vi "RCV CAN data FD.vi"() -> ()   [LabVIEW 2016]
doc: "This is a practical example of CAN_READ_FD.\nOn the left hand side of the BD is a disabled code section. One can enable this to log CAN data.\nThe potput of this disabled code segment is the error cluster.\nThan the selected channel will be initiatlized.\nOnce the initialisation is OK a timed while loop will be executed until CAN_READ_FD will signal an error.\nInside of the while loop is the CAN_READ_FD function.\nBuilding up an array of CAN mesages and timestamps is done while this loop executes.\nOnly the last message witch is naturaly empty, because the receive queue is empty, will be ignored.\nThe result is an array of received CAN messages."
uses:
  CAN Communication.llb/TPCANHandle.ctl
  CAN Communication.llb/TPCANTimestampFD.ctl
  CAN Communication.llb/CAN MSG Cluster.ctl
  CAN Communication.llb/TPCANParameter.ctl
  <vilib>/Platform/TimedLoop/XDataNode/timing_clust.ctl
  <vilib>/Platform/TimedLoop/XDataNode/nitl_modes.ctl
  <vilib>/Platform/TimedLoop/XDataNode/wakeup.ctl
  CAN Communication.llb/PCAN Get CHANNEL CONDITION.vi
  <vilib>/Platform/TimedLoop/XDataNode/XDataNode.xnode
  <vilib>/Platform/TimedLoop/XDataNode/XDNodeRunTimeDep.lvlib
  D:/Persoenliche_Daten/LabVIEW/VI.LIB/Peak/LV_basic FD Auslieferung/.LV Win32 VIs/Controls/LOG config.ctl
  D:/Persoenliche_Daten/LabVIEW/VI.LIB/Peak/LV_basic FD Auslieferung/.LV Win32 VIs/VIs/Set Value/PCAN Set LOG CONFIGURE.vi
  D:/Persoenliche_Daten/LabVIEW/VI.LIB/Peak/LV_basic FD Auslieferung/.LV Win32 VIs/VIs/Set Value/PCAN Set LOG LOCATION.vi
panel:
  out "TPCANMessageType out Strings":string
  out "CAN Data out":T1[](array[typedef]) {"MSG type" format="%x"; "ID" format="%.0x"}
  out "CAN Timestamp data out":T2[](array[typedef]) format="%x"
  in  "Release all channels first":bool
  in  "TPCANHandle":T3=enum."PCAN_USBBUS1  0x51"
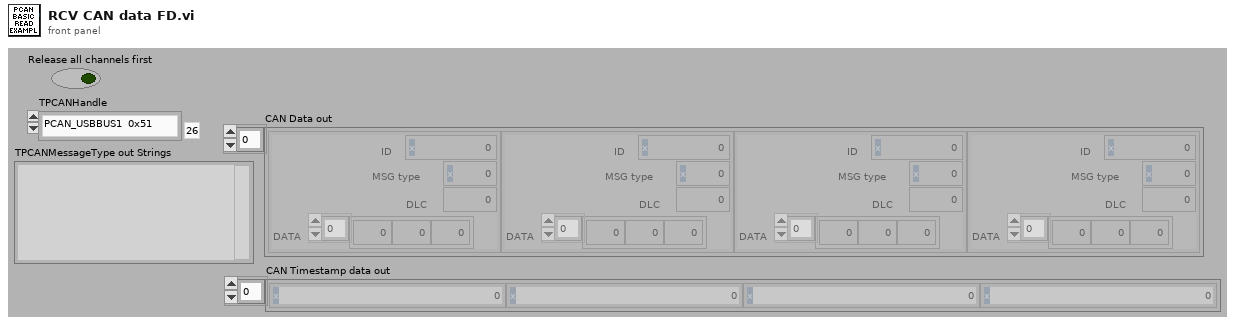
[diagram p1: front panel]
types:
  T1 = typedef "CAN MSG Cluster.ctl" = cluster{"ID":u32, "MSG type":u8, "DLC":u8, "DATA":u8[]}
  T2 = typedef "TPCANTimestampFD.ctl" = u64
  T3 = typedef "TPCANHandle.ctl" = enum16{"PCAN_NONEBUS  0x000", "PCAN_ISABUS1  0x21", "PCAN_ISABUS2  0x22", "PCAN_ISABUS3  0x23", "PCAN_ISABUS4  0x24", "PCAN_ISABUS5  0x25", "PCAN_ISABUS6  0x26", "PCAN_ISABUS7  0x27", "PCAN_ISABUS8  0x28", "PCAN_DNGBUS1  0x31", "PCAN_PCIBUS1  0x41", "PCAN_PCIBUS1  0x42", "PCAN_PCIBUS1  0x43", "PCAN_PCIBUS1  0x44", "PCAN_PCIBUS1  0x45", "PCAN_PCIBUS1  0x46", "PCAN_PCIBUS1  0x47", "PCAN_PCIBUS1  0x48", "PCAN_PCIBUS1  0x409", "PCAN_PCIBUS1  0x40A", "PCAN_PCIBUS1  0x40B", "PCAN_PCIBUS1  0x40C", "PCAN_PCIBUS1  0x40D", "PCAN_PCIBUS1  0x40E", "PCAN_PCIBUS1  0x40F", "PCAN_PCIBUS1  0x410", "PCAN_USBBUS1  0x51", "PCAN_USBBUS2  0x52", "PCAN_USBBUS3  0x53", "PCAN_USBBUS4  0x54", "PCAN_USBBUS5  0x55", "PCAN_USBBUS6  0x56", "PCAN_USBBUS7  0x57", "PCAN_USBBUS8  0x58", "PCAN_USBBUS9  0x509", "PCAN_USBBUS10  0x50A", "PCAN_USBBUS11  0x50B", "PCAN_USBBUS12  0x50C", "PCAN_USBBUS13  0x50D", "PCAN_USBBUS14  0x50E", "PCAN_USBBUS15  0x50F", "PCAN_USBBUS16  0x510", "PCAN_PCCBUS1  0x61", "PCAN_PCCBUS2  0x62", "PCAN_LANBUS1  0x801", "PCAN_LANBUS2  0x802", "PCAN_LANBUS3  0x803", "PCAN_LANBUS4  0x804", "PCAN_LANBUS5  0x805", "PCAN_LANBUS6  0x806", "PCAN_LANBUS7  0x807", "PCAN_LANBUS8  0x808", "PCAN_LANBUS9  0x809", "PCAN_LANBUS10  0x80A", "PCAN_LANBUS11  0x80B", "PCAN_LANBUS12  0x80C", "PCAN_LANBUS13  0x80D", "PCAN_LANBUS14  0x80E", "PCAN_LANBUS15  0x80F", "PCAN_LANBUS16  0x810"}
  T4 = typedef "TPCANParameter.ctl" = enum8{"Not Available", "PCAN device number", "PCAN 5-volt power", "PCAN receive event", "PCAN message filter", "PCAN API version", "PCAN channel version", "PCAN busoff autoreset", "PCAN listen-only", "PCAN log location", "PCAN log status", "PCAN log configure", "PCAN log text", "PCAN channel condition", "PCAN hardware name", "PCAN_RECEIVE_STATUS", "PCAN_CONTROLLER_NUMBER", "PCAN_TRACE_LOCATION ", "PCAN_TRACE_STATUS", "PCAN_TRACE_SIZE", "PCAN_TRACE_CONFIGURE", "PCAN_CHANNEL_IDENTIFYING", "PCAN_CHANNEL_FEATURES", "PCAN_SPEED_ADAPTING", "PCAN_BITRATE_INFO", "PCAN_BITRATE_INFO_FD", "PCAN_BUSSPEED_NOMINAL", "PCAN_BUSSPEED_DATA", "PCAN_IP_ADDRESS", "PCAN_LAN_SERVICE_STATUS", "PCAN_ALLOW_STATUS_FRAMES", "PCAN_ALLOW_RTR_FRAMES", "PCAN_ALLOW_ERROR_FRAMES", "PCAN_INTERFRAME_DELAY", "PCAN_ACCEPTANCE_FILTER_11BIT", "PCAN_ACCEPTANCE_FILTER_29BIT", "PCAN_IO_DIGITAL_CONFIGURATION", "PCAN_IO_DIGITAL_VALUE", "PCAN_IO_DIGITAL_SET", "PCAN_IO_DIGITAL_CLEAR", "PCAN_IO_ANALOG_VALUE"}
  T5 = typedef "PCAN BASIC FD.lvlib/LOG config.ctl" = u32
  T6 = typedef "PCAN BASIC FD.lvlib/TPCANHandle.ctl" = enum16{"PCAN_NONEBUS  0x000", "PCAN_ISABUS1  0x21", "PCAN_ISABUS2  0x22", "PCAN_ISABUS3  0x23", "PCAN_ISABUS4  0x24", "PCAN_ISABUS5  0x25", "PCAN_ISABUS6  0x26", "PCAN_ISABUS7  0x27", "PCAN_ISABUS8  0x28", "PCAN_DNGBUS1  0x31", "PCAN_PCIBUS1  0x41", "PCAN_PCIBUS1  0x42", "PCAN_PCIBUS1  0x43", "PCAN_PCIBUS1  0x44", "PCAN_PCIBUS1  0x45", "PCAN_PCIBUS1  0x46", "PCAN_PCIBUS1  0x47", "PCAN_PCIBUS1  0x48", "PCAN_PCIBUS1  0x409", "PCAN_PCIBUS1  0x40A", "PCAN_PCIBUS1  0x40B", "PCAN_PCIBUS1  0x40C", "PCAN_PCIBUS1  0x40D", "PCAN_PCIBUS1  0x40E", "PCAN_PCIBUS1  0x40F", "PCAN_PCIBUS1  0x410", "PCAN_USBBUS1  0x51", "PCAN_USBBUS2  0x52", "PCAN_USBBUS3  0x53", "PCAN_USBBUS4  0x54", "PCAN_USBBUS5  0x55", "PCAN_USBBUS6  0x56", "PCAN_USBBUS7  0x57", "PCAN_USBBUS8  0x58", "PCAN_USBBUS9  0x509", "PCAN_USBBUS10  0x50A", "PCAN_USBBUS11  0x50B", "PCAN_USBBUS12  0x50C", "PCAN_USBBUS13  0x50D", "PCAN_USBBUS14  0x50E", "PCAN_USBBUS15  0x50F", "PCAN_USBBUS16  0x510", "PCAN_PCCBUS1  0x61", "PCAN_PCCBUS2  0x62", "PCAN_LANBUS1  0x81", "PCAN_LANBUS2  0x82", "PCAN_LANBUS3  0x83", "PCAN_LANBUS4  0x84", "PCAN_LANBUS5  0x85", "PCAN_LANBUS6  0x86", "PCAN_LANBUS7  0x87", "PCAN_LANBUS8  0x88", "PCAN_LANBUS9  0x809", "PCAN_LANBUS10  0x80A", "PCAN_LANBUS11  0x80B", "PCAN_LANBUS12  0x80C", "PCAN_LANBUS13  0x80D", "PCAN_LANBUS14  0x80E", "PCAN_LANBUS15  0x80F", "PCAN_LANBUS16  0x810"}
  T7 = typedef "Channel Availability.ctl" = enum16{"PCAN_CHANNEL_UNAVAILABLE", "PCAN_CHANNEL_AVAILABLE", "PCAN_CHANNEL_OCCUPIED"}
  T8 = typedef "XDNodeRunTimeDep.lvlib/timing_clust.ctl" = cluster{"Expected End [f-1]":u64, "Actual End [f-1]":u64, "Finished Late? [f-1]":bool, "Expected End [i-1]":u64, "Actual End [i-1]":u64, "Finished Late? [i-1]":bool, "Expected Start [i]":u64, "Actual Start [i]":u64, "Expected Start [f]":u64, "Actual Start [f]":u64, "Source Name":string, "Structure Name":string, "Period":i64, "Deadline":i64, "Offset":i64, "Start":i64, "Priority":i32, "Timeout":i32, "Mode":T9, "Wakeup Reason":T10, "Error":errorcluster, "Source Type":string, "Secondary Source Type":string, "Global End Time":u64, "Global Start Time":u64, "Frame Duration":u64, "Iteration Duration":u64, "Assigned CPU":i32, "I/O Scan Engine Mode":u32}
  T9 = typedef "XDNodeRunTimeDep.lvlib/nitl_modes.ctl" = enum32{"No Change", "Process missed periods, maintain original phase", "Discard missed periods, maintain original phase", "Process missed periods, ignore original phase", "Discard missed periods, ignore original phase"}
  T10 = typedef "XDNodeRunTimeDep.lvlib/wakeup.ctl" = enum32{"Normal", "Aborted", "Asynchronous wakeup", "Timing source error", "Timed loop error", "Timeout"}
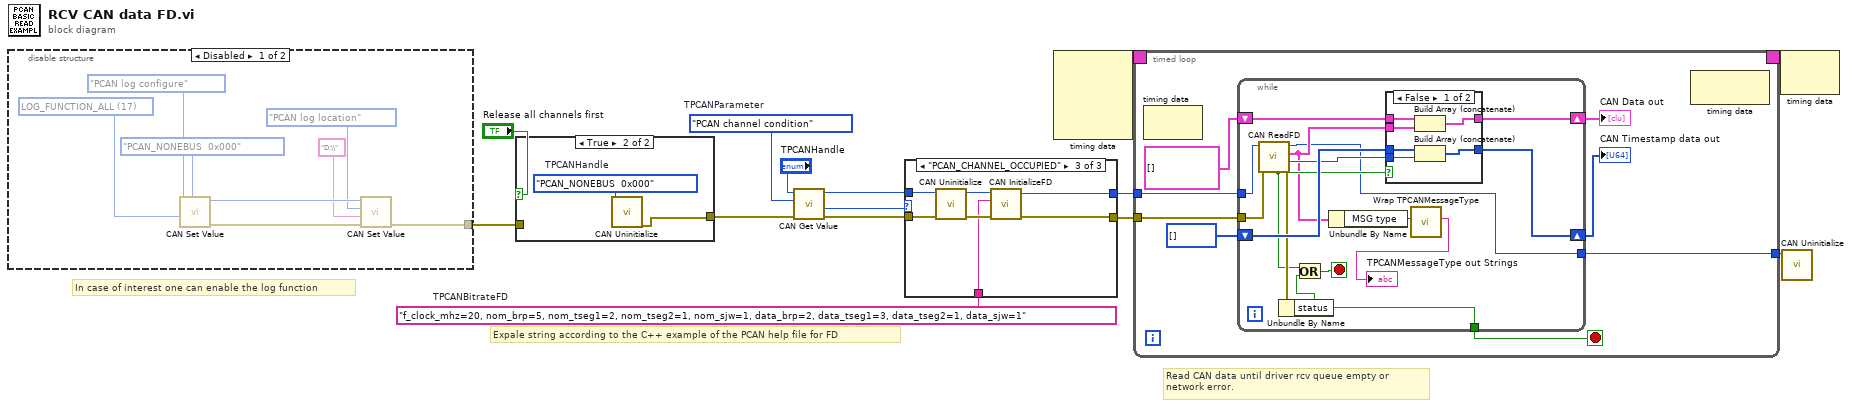
[diagram p0: block diagram]
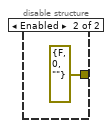
[diagram p3: hidden frame]
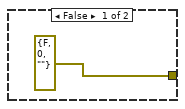
[diagram p4: hidden frame]
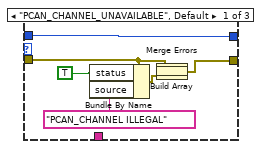
[diagram p5: hidden frame]
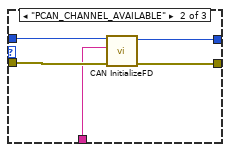
[diagram p6: hidden frame]
diagram:
  w9 = "f_clock_mhz=20, nom_brp=5, nom_tseg1=2, nom_tseg2=1, nom_sjw=1, data_brp=2, data_tseg1=3, data_tseg2=1, data_sjw=1"  # TPCANBitrateFD
  w14 = TPCANParameter."PCAN channel condition"  # TPCANParameter
  # "In case of interest one can enable the log function"
  # "Read CAN data until driver rcv queue empty or\nnetwork error."
  # "Expale string according to the C++ example of the PCAN help file for FD"
  n1 = disable-structure shown="Disabled" {
    disable-tunnel: [w15 errorcluster {"status"=FALSE, "code"=0, "source"=""} ("error out")] -> w6
    frame Disabled {
      w16 = T5 17 items=["LOG_FUNCTION_DEFAULT", "LOG_FUNCTION_ENTRY", "LOG_FUNCTION_PARAMETERS", "Not available", "LOG_FUNCTION_LEAVE", "Not available", "Not available", "Not available", "LOG_FUNCTION_WRITE", "Not available", "Not available", "Not available", "Not available", "Not available", "Not available", "Not available", "LOG_FUNCTION_READ", "LOG_FUNCTION_ALL"] ("LOG config")
      n2 = call-poly "CAN Set Value.vi"("LOG config"=w16, "TPCANParameter"=TPCANParameter."PCAN log configure", "TPCANHandle"=TPCANHandle."PCAN_NONEBUS  0x000") -> ("error out"=w21:errorcluster, "TPCANHandle out"=w20:T6)  [unwired: 7 in]
      n3 = call-poly "CAN Set Value.vi"("error in (no error)"=w21, "LOG LOCATION (path string)"="D:\\", "Parameter"=TPCANParameter."PCAN log location", "TPCANHandle"=w20) -> ("error out"=w15:errorcluster)  [unwired: 6 in, 1 out]
    }
    frame Enabled {
    }
  }
  n4 = case shown="True" "Release all channels first" {
    tunnel: [errorcluster {"status"=FALSE, "code"=0, "source"=""} ("error out") w26] -> w7
    tunnel: w6 -> [_ _]
    frame False {
    }
    frame True {
      w25 = TPCANHandle."PCAN_NONEBUS  0x000"  # TPCANHandle
      n5 = call "CAN Uninitialize.vi"("TPCANHandle"=w25) -> ("error out"=w26:errorcluster)  [unwired: 8 in, 2 out]
    }
  }
  n6 = call-poly "CAN Get Value.vi"("error in (no error)"=w7, "TPCANParameter"=w14, "TPCANHandle"="TPCANHandle") -> ("error out"=w12:errorcluster, "Channel condition"=w11:T7, "TPCANHandle out"=w13:T3)  [unwired: 6 in]
  n7 = case shown="\"PCAN_CHANNEL_OCCUPIED\"" w11 {
    tunnel: [w32 w38 w42] -> w3
    tunnel: w13 -> [w33 w37 w44]
    tunnel: w12 -> [w31 w36 w45]
    tunnel: [w33 w35 w40] -> w2
    tunnel: w9 -> [_ w34 w39]
    frame "PCAN_CHANNEL_UNAVAILABLE", Default {
      n8 = Bundle By Name(cluster=w31, "status"=TRUE, "source"="PCAN_CHANNEL ILLEGAL") -> (w28:errorcluster)
      n9 = Build Array(w31, w28) -> (w27:errorcluster[])
      n10 = Merge Errors(w27) -> (w32:errorcluster)
    }
    frame "PCAN_CHANNEL_AVAILABLE" {
      n11 = call "CAN InitializeFD.vi"("error in (no error)"=w36, "TPCANBitrateFD"=w34, "TPCANHandle"=w37) -> ("error out"=w38:errorcluster, "TPCANHandle out"=w35:T3)  [unwired: 5 in, 2 out]
    }
    frame "PCAN_CHANNEL_OCCUPIED" {
      n12 = call "CAN Uninitialize.vi"("error in (no error)"=w45, "TPCANHandle"=w44) -> ("error out"=w43:errorcluster, "TPCANHandle out"=w41:T3)  [unwired: 7 in, 1 out]
      n13 = call "CAN InitializeFD.vi"("error in (no error)"=w43, "TPCANBitrateFD"=w39, "TPCANHandle"=w41) -> ("error out"=w42:errorcluster, "TPCANHandle out"=w40:T3)  [unwired: 5 in, 2 out]
    }
  }
  n14 = node-c288() -> (w5:T8)  [unwired: 4 in]
  n15 = timed-loop {
    timing: w5 -> [_]
    timing-out: [_] -> w4
    tunnel: w2 -> [w53]
    tunnel: w3 -> [w52]
    tunnel: [w46] -> w1
    stop <- w51 stop-if-true
    n16 = node-c288() -> ()  [unwired: 1 in, 1 out]
    n17 = while {
      tunnel: w53 -> [w62]
      tunnel: w52 -> [w61]
      tunnel: [w67] -> w51
      shift-right: [w65] -> w50
      shift-left: T1[] [] -> [w66]
      shift-right: [w63] -> w47
      shift-left: u64[] [] -> [w64]
      tunnel: [w54] -> w46
      stop <- w68 stop-if-true
      n18 = call "CAN ReadFD.vi"("error in (no error)"=w61, "TPCANHandle"=w62) -> ("error out"=w59:errorcluster, "TPCANTimestamp out"=w60:T2, "CAN_Message out"=w55:T1, "TPCANHandle out"=w54:T3, "rcv queue empty"=w58:bool)  [unwired: 5 in]
      n19 = Unbundle By Name(w59) -> ("status"=w67:bool)
      n20 = Or(x=w58, y=w67) -> (x .or. y?=w68:bool)
      n21 = Unbundle By Name(w55) -> ("MSG type"=w56:u8)
      n22 = case shown="False" w58 {
        tunnel: w66 -> [w74 w76]
        tunnel: [w73 w76] -> w65
        tunnel: w55 -> [w72 _]
        tunnel: w64 -> [w71 w75]
        tunnel: w60 -> [w70 _]
        tunnel: [w69 w75] -> w63
        frame False {
          n23 = Build Array (concatenate)(w74, w72) -> (w73:T1[])
          n24 = Build Array (concatenate)(w71, w70) -> (w69:T2[])
        }
        frame True {
        }
      }
      n25 = call "Wrap TPCANMessageType.vi"("TPCANMessageType Numeric"=w56) -> ("TPCANMessageType out Strings"=→"TPCANMessageType out Strings":string)  [unwired: 9 in, 1 out]
    }
    "CAN Data out" <- w50
    "CAN Timestamp data out" <- w47
    n26 = node-c288() -> ()  [unwired: 1 in, 1 out]
  }
  n27 = node-c288(w4) -> ()  [unwired: 1 out]
  n28 = call "CAN Uninitialize.vi"("TPCANHandle"=w1) -> ()  [unwired: 8 in, 3 out]
